vi "New SSE Client.vi"(7 "Last Event ID (None)":string, 8 "error in (no error)":errorcluster, 10 "SSE Client":refnum<class "SSE Client.lvclass">, 11 "SSE Manager in":refnum<class "SSE Manager.lvclass">) -> (0 "error out":errorcluster, 3 "SSE Manager out":refnum<class "SSE Manager.lvclass">)   [LabVIEW 2020, in "HTTP Server.lvlib" / "SSE Manager.lvclass"]
uses:
  SSE Manager.lvclass
  SSE Client/SSE Client.lvclass
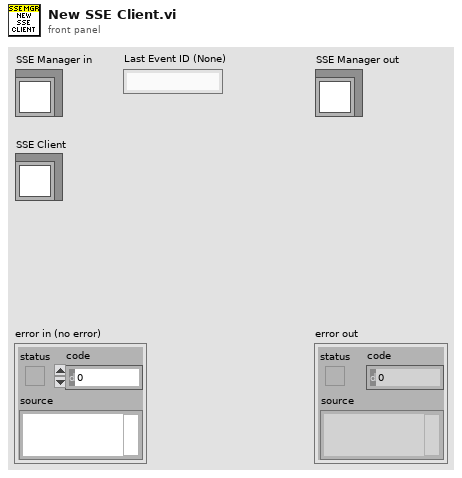
[diagram p1: front panel]
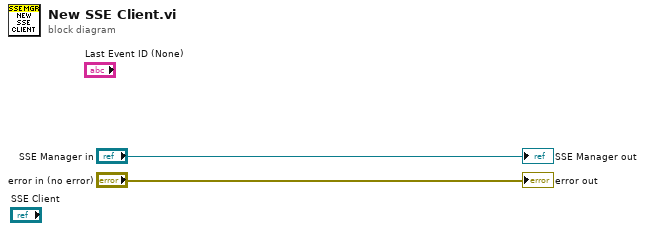
[diagram p0: block diagram]
diagram:
  "error out" <- "error in (no error)"
  "SSE Manager out" <- "SSE Manager in"
